vi "get_array_position_with_saturation.vi"(9 "array size":i32, 11 "array position":i32) -> (3 "array positions":i32[](array[numeric]))   [LabVIEW 2010]
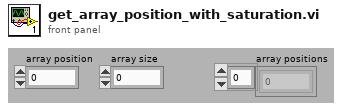
[diagram p1: front panel]
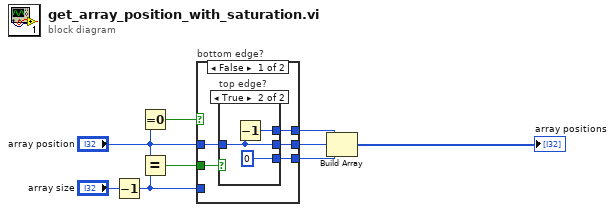
[diagram p0: block diagram]
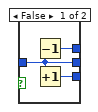
[diagram p2: hidden frame]
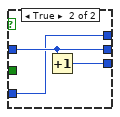
[diagram p3: hidden frame]
diagram:
  n1 = Decrement(x="array size") -> (x-1=w1:i32)
  n2 = Equal To 0?(x="array position") -> (x = 0?=w3:bool)
  n3 = Equal?(x="array position", y=w1) -> (x = y?=w4:bool)
  n4 = case "bottom edge?" shown="False" w3 {
    tunnel: "array position" -> [w14 w23]
    tunnel: [w10 w23] -> w7
    tunnel: [w13 w22] -> w8
    tunnel: [w12 w21] -> w6
    tunnel: w1 -> [_ w21]
    tunnel: w4 -> [w11 _]
    frame False {
      n5 = case "top edge?" shown="True" w11 {
        tunnel: w14 -> [w15 w18]
        tunnel: [w17 0] -> w13
        tunnel: [w16 w20] -> w12
        tunnel: [w15 w18] -> w10
        frame False {
          n6 = Decrement(x=w15) -> (x-1=w16:i32)
          n7 = Increment(x=w15) -> (x+1=w17:i32)
        }
        frame True {
          n8 = Decrement(x=w18) -> (x-1=w20:i32)
        }
      }
    }
    frame True {
      n9 = Increment(x=w23) -> (x+1=w22:i32)
    }
  }
  n10 = Build Array(w6, w7, w8) -> (→"array positions":i32[])
